vi "Instrument.PPMS2.Read Configuration File.vi"(8 "error in (no error)":errorcluster, 11 "instrument.PPMS2 in":refnum<class "instrument.PPMS2.lvclass">) -> (0 "error out":errorcluster, 3 "instrument.PPMS2 out":refnum<class "instrument.PPMS2.lvclass">)   [LabVIEW 2016, in "instrument.PPMS2.lvclass"]
uses:
  instrument.PPMS2.lvclass
  C:/Program Files (x86)/National Instruments/LabVIEW 2016/user.lib/LevyLab/Levylab Instruments/SMOs/Instrument/Instrument.lvclass
  <userlib>/LevyLab/Levylab Instruments/SMOs/Instrument/Instrument.lvclass/Instrument.ctl
  instrument.PPMS2.lvclass/instrument.PPMS2.ctl
  <userlib>/LevyLab/Levylab Instruments/SMOs/Configuration/Configuration.lvclass
  <userlib>/LevyLab/Levylab Instruments/SMOs/Instrument/Instrument.lvclass
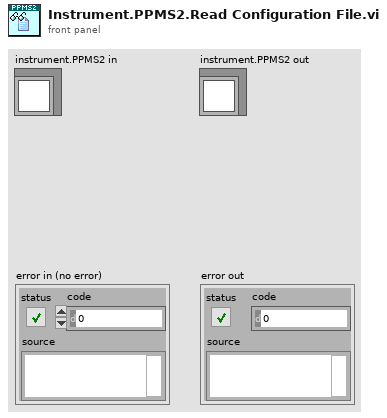
[diagram p1: front panel]
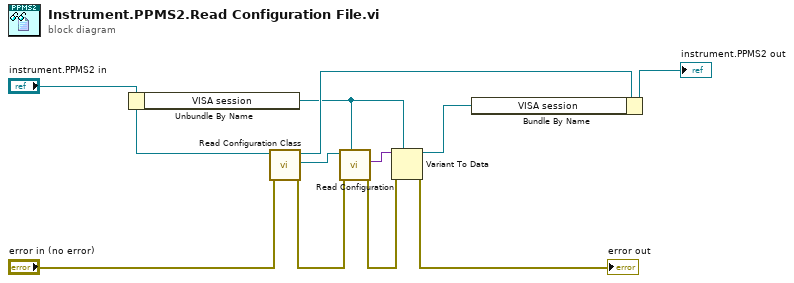
[diagram p0: block diagram]
diagram:
  n1 = Unbundle By Name("instrument.PPMS2 in") -> ("VISA session"=w3:refnum<visa-resource-name>)
  n2 = call <userlib>:"Read Configuration Class.vi"("error in (no error)"="error in (no error)", "Instrument in"="instrument.PPMS2 in") -> ("error out"=w8:errorcluster, "Configuration.lvclass"=w9:refnum<class "Configuration.lvclass">, "Instrument out"=w6:refnum<class "instrument.PPMS2.lvclass">)  [unwired: 7 in]
  n3 = call <userlib>:"Read Configuration.vi"("INI Fomatted Cluster Type"=w3, "error in (no error)"=w8, "Configuration in"=w9) -> ("error out"=w10:errorcluster, "Configuration"=w11:variant)  [unwired: 6 in, 1 out]
  n4 = Variant To Data(error in=w10, type=w3, Variant=w11) -> (data=w1:refnum<visa-resource-name>, error out=→"error out":errorcluster)
  n5 = Bundle By Name(cluster=w6, "VISA session"=w1) -> (→"instrument.PPMS2 out":refnum<class "instrument.PPMS2.lvclass">)
